vi "List Tester.vi"() -> ()   [LabVIEW 2016]
uses:
  Horizontal MenuList.xctl
panel:
  in  "HorizontalList":i32(xcontrol)
  in  "List Val Controller":i32
  out "Indicator List":i32(xcontrol)
  in  "Item Names":string[](array[string])=["Welcome", "System", "Data Viewer", "Settings", "Help"]
  out "Count":i32=5
  # "List as an indicator"
  # "Edit the numeric control. The list will update its selection. Out of bounds value\nare coerced."
  # "Edit the array above. The list at the top of the FP \nwill update accordingly."
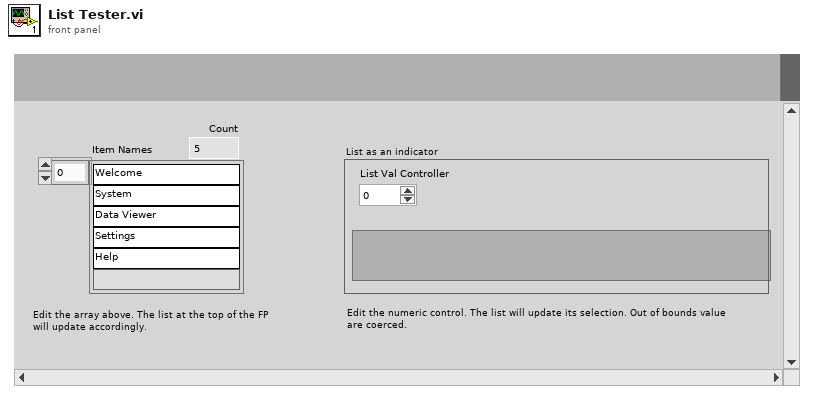
[diagram p1: front panel]
types:
  T1 = cluster{"Font Name:":string, "Size":i16, "Strikeout?":bool, "Italic?":bool, "Underline?":bool, "Outline?":bool, "Shadow?":bool, "Bold?":bool}
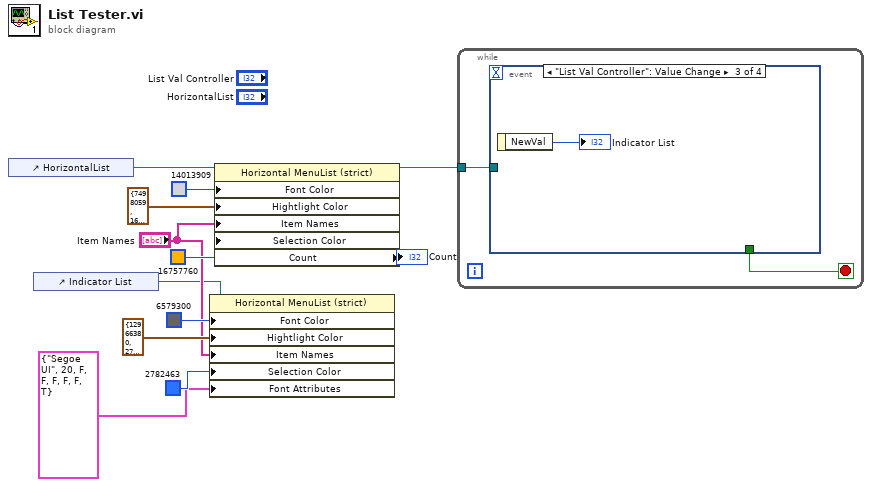
[diagram p0: block diagram]
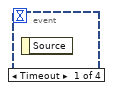
[diagram p2: hidden frame]
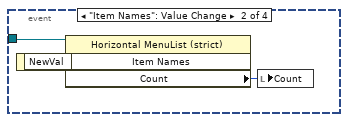
[diagram p3: hidden frame]
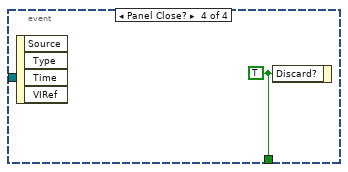
[diagram p4: hidden frame]
diagram:
  n1 = control-ref of="HorizontalList"() -> (w1:refnum<vi>)
  n2 = control-ref of="Indicator List"() -> (w2:refnum<vi>)
  n3 = property class="Horizontal MenuList (strict)"(reference=w2, "Font Color"=u32 6579300 ("Back"), "Hightlight Color"=cluster{"Back":u32, "Edge":u32} {"Back"=12966380, "Edge"=2782463}, "Item Names"="Item Names", "Selection Color"=u32 2782463 ("Back"), "Font Attributes"=T1 {"Font Name:"="Segoe UI", "Size"=20, "Strikeout?"=FALSE, "Italic?"=FALSE, "Underline?"=FALSE, "Outline?"=FALSE, "Shadow?"=FALSE, "Bold?"=TRUE}) -> ()  [unwired: 1 in, 2 out]
  n4 = property class="Horizontal MenuList (strict)"(reference=w1, "Font Color"=u32 14013909 ("Back"), "Hightlight Color"=cluster{"Back":u32, "Edge":u32} {"Back"=7498059, "Edge"=16757760}, "Item Names"="Item Names", "Selection Color"=u32 16757760 ("Back")) -> (reference out=w9:refnum<vi>, "Count"=→"Count":i16)  [unwired: 1 in, 1 out]
  n5 = while {
    tunnel: w9 -> [w13]
    stop <- w14 stop-if-true
    n6 = event shown="[2] \"List Val Controller\": Value Change" {
      selector: _ -> [_ _ _ _]
      dyn-events: _ -> [_ _ _ _]
      timeout: _ -> [_ _ _ _]
      tunnel: [_ _ _ w19] -> w14
      tunnel: w13 -> [_ w17 _ _]
      event Timeout {
        n7 = event-data() -> ()  [unwired: 1 in, 1 out]
      }
      event "Item Names": Value Change {
        n8 = event-data() -> ("NewVal"=w16:string[])  [unwired: 1 in]
        n9 = property class="Horizontal MenuList (strict)"(reference=w17, "Item Names"=w16) -> ("Count"=w15:i16)  [unwired: 1 in, 2 out]
        n10 = local write "Count"(w15) -> ()
      }
      event "List Val Controller": Value Change {
        n11 = event-data() -> ("NewVal"=→"Indicator List":i32)  [unwired: 1 in]
      }
      event Panel Close? {
        w19 = TRUE ("Discard?")
        n12 = event-data() -> ()  [unwired: 1 in, 4 out]
        n13 = event-data("Discard?"=w19) -> ()  [unwired: 1 in, 1 out]
      }
    }
  }
